vi "Translator.vi"(0 "Input":variant, 11 "error in (no error)":errorcluster) -> (4 "Output":variant, 15 "error out":errorcluster)   [LabVIEW 2014, in "Complex Numbers Static.lvlib"]
doc: "An example of how to create the Translator to convert the LabVIEW VIs to Arduino C code."
uses:
  Complex Numbers Static.lvlib
panel:
  out "Outputs":string[](array[string])
  out "Inputs":string[](array[string])
  out "Output Datatypes":string[](array[string])
  out "Input Datatypes":string[](array[string])
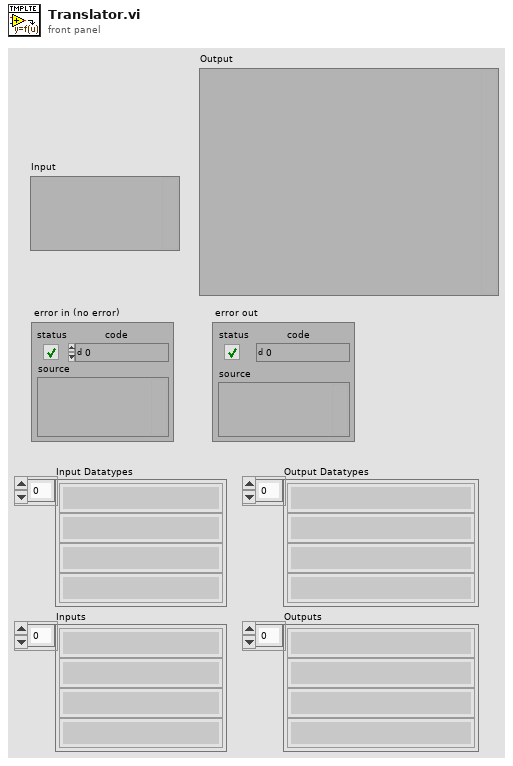
[diagram p1: front panel]
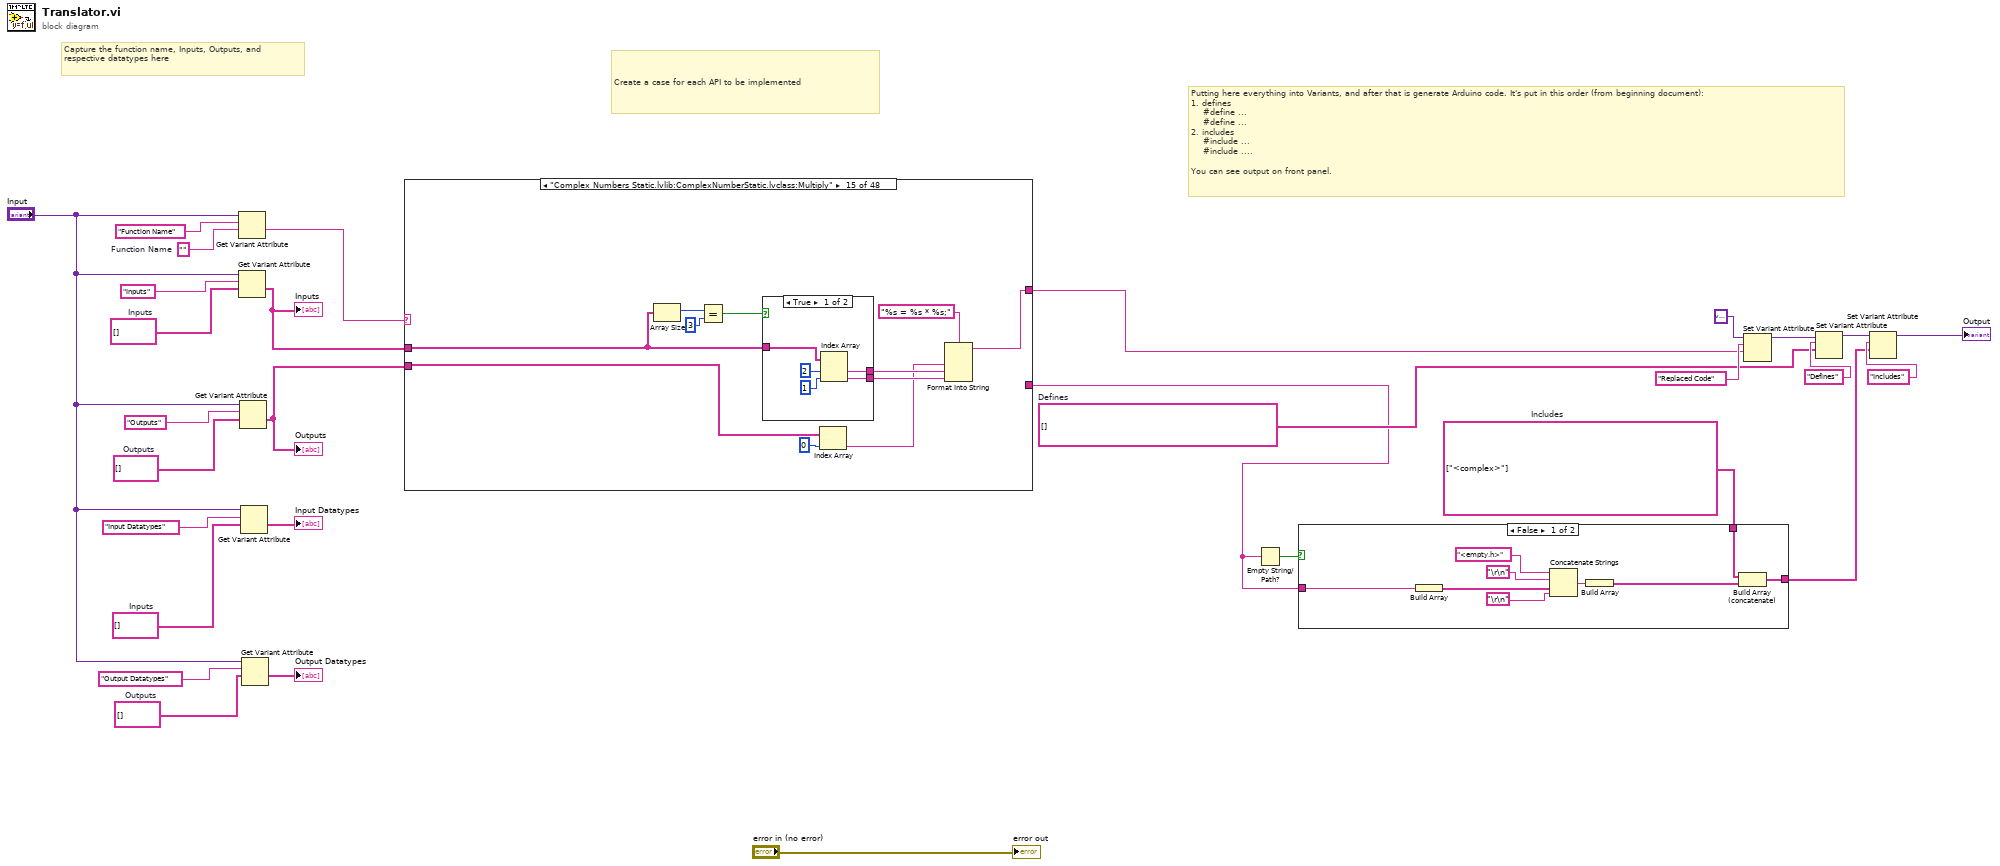
[diagram p0: block diagram]
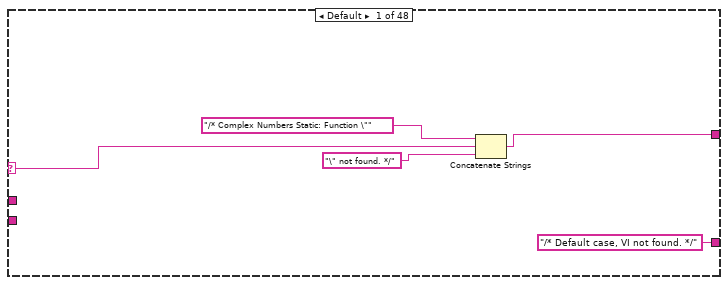
[diagram p3: hidden frame]
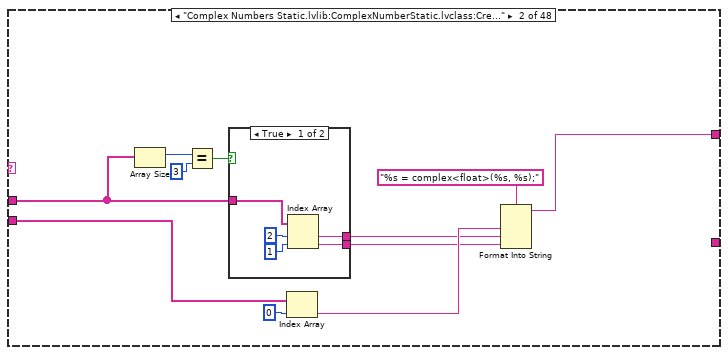
[diagram p4: hidden frame]
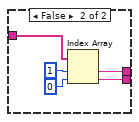
[diagram p5: hidden frame]
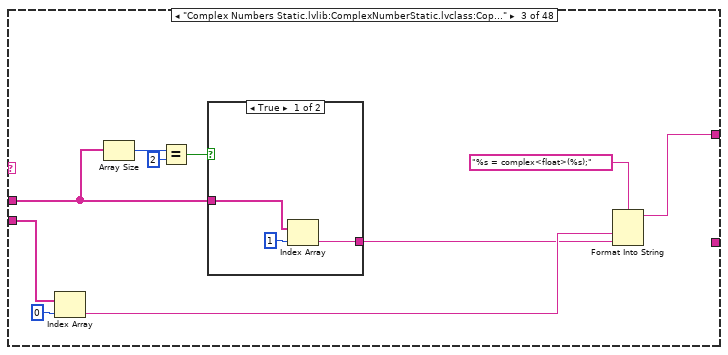
[diagram p6: hidden frame]
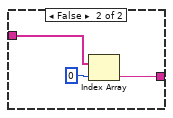
[diagram p7: hidden frame]
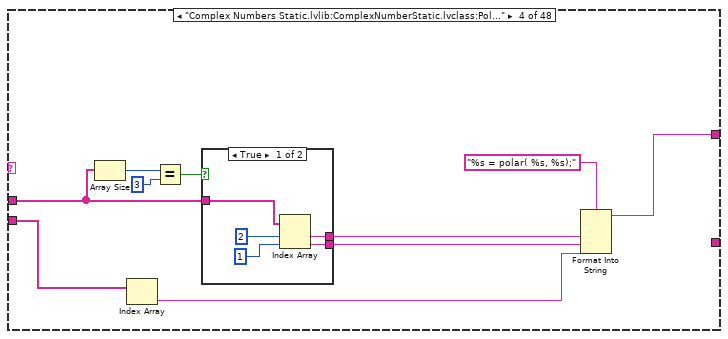
[diagram p8: hidden frame]
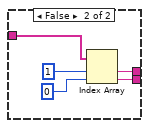
[diagram p9: hidden frame]
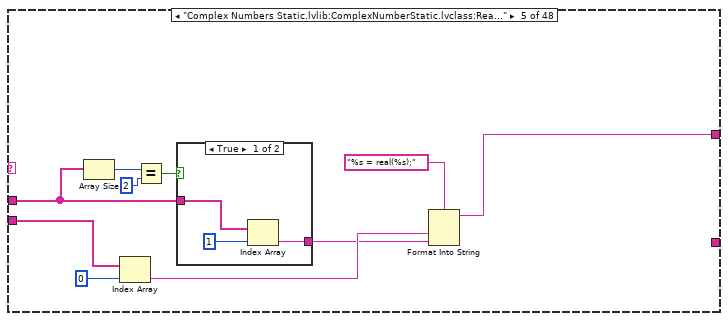
[diagram p10: hidden frame]
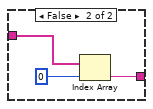
[diagram p11: hidden frame]
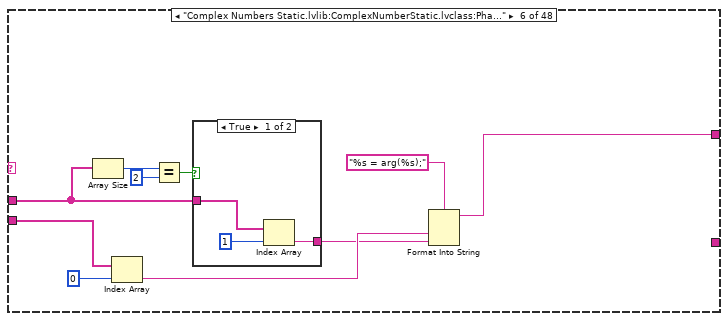
[diagram p12: hidden frame]
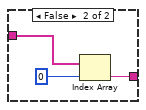
[diagram p13: hidden frame]
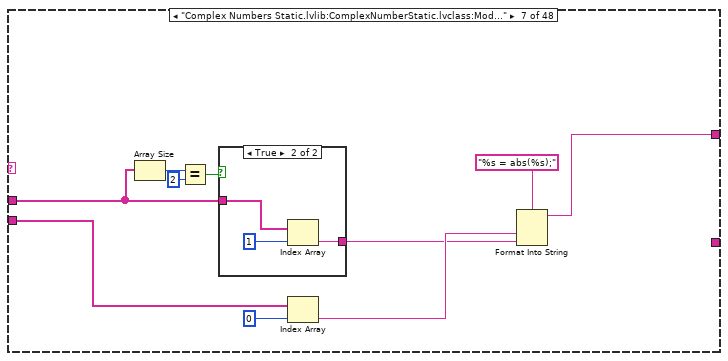
[diagram p14: hidden frame]
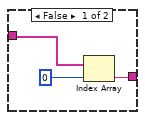
[diagram p15: hidden frame]
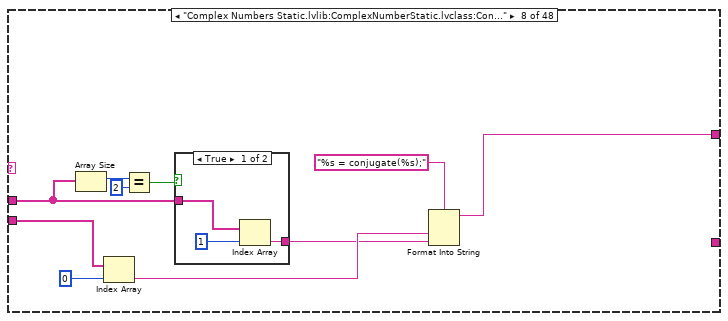
[diagram p16: hidden frame]
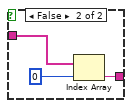
[diagram p17: hidden frame]
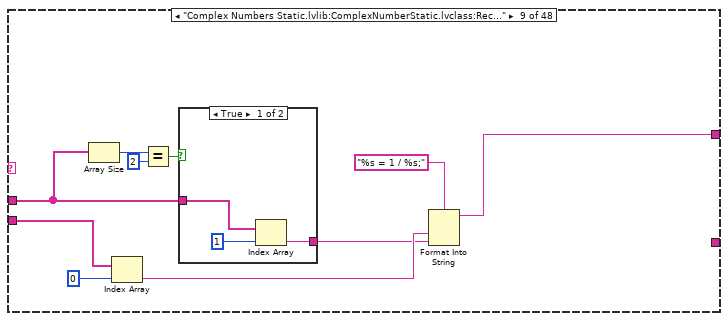
[diagram p18: hidden frame]
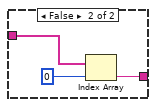
[diagram p19: hidden frame]
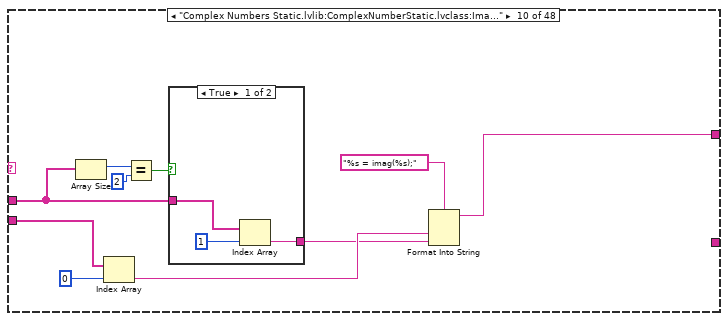
[diagram p20: hidden frame]
diagram:
  w4 = string[] []  # Defines
  w19 = string[] []  # Outputs
  w20 = string[] []  # Inputs
  w1 = string[] ["<complex>"]  # Includes
  w26 = string[] []  # Outputs
  w27 = string[] []  # Inputs
  w28 = ""  # Function Name
  # "Capture the function name, Inputs, Outputs, and respective datatypes here"
  # "Putting here everything into Variants, and after that is generate Arduino code. It's put in this order (from beginning document):\n1. defines\n    #define ...\n    #define ...\n2. includes\n    #include ...\n    #include ....\n\nYou can see output on front panel."
  # "Create a case for each API to be implemented"
  n1 = Get Variant Attribute(Variant="Input", name="Function Name", default value (empty Variant)=w28) -> (value=w10:string)  [unwired: 1 in, 3 out]
  n2 = Get Variant Attribute(Variant="Input", name="Inputs", default value (empty Variant)=w27) -> (value=w9:string[])  [unwired: 1 in, 3 out]
  "Inputs" <- w9
  n3 = Get Variant Attribute(Variant="Input", name="Outputs", default value (empty Variant)=w26) -> (value=w8:string[])  [unwired: 1 in, 3 out]
  "Outputs" <- w8
  n4 = Get Variant Attribute(Variant="Input", name="Input Datatypes", default value (empty Variant)=w20) -> (value=→"Input Datatypes":string[])  [unwired: 1 in, 3 out]
  n5 = Get Variant Attribute(Variant="Input", name="Output Datatypes", default value (empty Variant)=w19) -> (value=→"Output Datatypes":string[])  [unwired: 1 in, 3 out]
  n6 = case shown="\"Complex Numbers Static.lvlib:ComplexNumberStatic.lvclass:Multiply\"" w10 {
    selector: w10 -> [w33 _ _ _ _ _ _ _ _ _ _ _ _ _ _ _ _ _ _ _ _ _ _ _ _ _ _ _ _ _ _ _ _ _ _ _ _ _ _ _ _ _ _ _ _ _ _ _]
    tunnel: w9 -> [_ w37 w57 w74 w94 w112 w128 w142 w158 w174 w191 w197 w218 w240 w260 w281 w302 w325 w339 w356 w377 w393 w410 w426 w445 w461 w478 w493 w509 w525 w541 w557 w573 w589 w605 w623 w637 w654 w670 w685 w701 w717 w733 w749 w766 w782 _ w813]
    tunnel: w8 -> [_ w43 w63 w77 w99 w115 w131 w147 w163 w179 w194 w204 w225 w246 w267 w289 w310 w330 w346 w363 w383 w399 w415 w432 w452 w468 w484 w500 w516 w532 w548 w564 w580 w596 w612 w622 w644 w660 w676 w692 w708 w724 w740 w756 w772 w788 w797 w819]
    tunnel: [w31 w42 w62 w82 w101 w117 w133 w149 w165 w181 w193 w202 w224 w245 w265 w288 w309 w329 w345 w362 w382 w398 w414 w431 w451 w467 w483 w499 w515 w531 w547 w563 w579 w595 w611 w621 w643 w659 w675 w691 w707 w723 w739 w755 w771 w787 w803 w818] -> w7
    tunnel: ["/* Default case, VI not found. */" ("name") _ _ _ _ _ _ _ _ _ _ _ _ _ _ _ _ _ _ _ _ _ _ _ _ _ _ _ _ _ _ _ _ _ _ _ _ _ _ _ _ _ _ _ _ _ _ _] -> w3
    frame Default {
      n7 = Concatenate Strings("/* Complex Numbers Static: Function \"" ("string"), w33, "\" not found. */" ("string")) -> (w31:string)
    }
    frame "Complex Numbers Static.lvlib:ComplexNumberStatic.lvclass:Create" {
      n8 = Array Size(array=w37) -> (size(s)=w38:i32)
      n9 = Equal?(x=w38, y=3) -> (x = y?=w39:bool)
      n10 = case shown="True" w39 {
        tunnel: w37 -> [w50 w55]
        tunnel: [w49 w54] -> w41
        tunnel: [w48 w53] -> w40
        frame True {
          n11 = Index Array(array=w50, index #1=2 ("index"), index #2=1 ("index")) -> (element #1=w49:string, element #2=w48:string)
        }
        frame False {
          n12 = Index Array(array=w55, index #1=1 ("index"), index #2=0 ("index")) -> (element #1=w54:string, element #2=w53:string)
        }
      }
      n13 = Index Array(array=w43, index=0) -> (element=w45:string)
      n14 = Format Into String(format string="%s = complex<float>(%s, %s);", w45, w41, w40) -> (resulting string=w42:string)  [unwired: 2 in, 1 out]
    }
    frame "Complex Numbers Static.lvlib:ComplexNumberStatic.lvclass:Copy" {
      n15 = Index Array(array=w63, index=0) -> (element=w65:string)
      n16 = Array Size(array=w57) -> (size(s)=w60:i32)
      n17 = Equal?(x=w60, y=2) -> (x = y?=w59:bool)
      n18 = case shown="True" w59 {
        tunnel: w57 -> [w68 w71]
        tunnel: [w67 w70] -> w61
        frame True {
          n19 = Index Array(array=w68, index=1) -> (element=w67:string)
        }
        frame False {
          n20 = Index Array(array=w71, index=0) -> (element=w70:string)
        }
      }
      n21 = Format Into String(format string="%s = complex<float>(%s);", w65, w61) -> (resulting string=w62:string)  [unwired: 2 in, 1 out]
    }
    frame "Complex Numbers Static.lvlib:ComplexNumberStatic.lvclass:Polar" {
      n22 = Array Size(array=w74) -> (size(s)=w79:i32)
      n23 = Index Array(array=w77) -> (element=w76:string)  [unwired: 1 in]
      n24 = Equal?(x=w79, y=3) -> (x = y?=w75:bool)
      n25 = case shown="True" w75 {
        tunnel: w74 -> [w86 w91]
        tunnel: [w84 w89] -> w81
        tunnel: [w83 w88] -> w80
        frame True {
          n26 = Index Array(array=w86, index #1=2 ("index"), index #2=1 ("index")) -> (element #1=w84:string, element #2=w83:string)
        }
        frame False {
          n27 = Index Array(array=w91, index #1=1 ("index"), index #2=0 ("index")) -> (element #1=w89:string, element #2=w88:string)
        }
      }
      n28 = Format Into String(format string="%s = polar( %s, %s);", w81, w80, w76) -> (resulting string=w82:string)  [unwired: 2 in, 1 out]
    }
    frame "Complex Numbers Static.lvlib:ComplexNumberStatic.lvclass:Real" {
      n29 = Array Size(array=w94) -> (size(s)=w95:i32)
      n30 = Index Array(array=w99, index=0) -> (element=w98:string)
      n31 = Equal?(x=w95, y=2) -> (x = y?=w96:bool)
      n32 = case shown="True" w96 {
        tunnel: w94 -> [w104 w107]
        tunnel: [w103 w106] -> w97
        frame True {
          n33 = Index Array(array=w104, index=1) -> (element=w103:string)
        }
        frame False {
          n34 = Index Array(array=w107, index=0) -> (element=w106:string)
        }
      }
      n35 = Format Into String(format string="%s = real(%s);", w98, w97) -> (resulting string=w101:string)  [unwired: 2 in, 1 out]
    }
    frame "Complex Numbers Static.lvlib:ComplexNumberStatic.lvclass:Phase" {
      n36 = Array Size(array=w112) -> (size(s)=w110:i32)
      n37 = Index Array(array=w115, index=0) -> (element=w114:string)
      n38 = Equal?(x=w110, y=2) -> (x = y?=w111:bool)
      n39 = case shown="True" w111 {
        tunnel: w112 -> [w120 w123]
        tunnel: [w119 w122] -> w113
        frame True {
          n40 = Index Array(array=w120, index=1) -> (element=w119:string)
        }
        frame False {
          n41 = Index Array(array=w123, index=0) -> (element=w122:string)
        }
      }
      n42 = Format Into String(format string="%s = arg(%s);", w114, w113) -> (resulting string=w117:string)  [unwired: 2 in, 1 out]
    }
    frame "Complex Numbers Static.lvlib:ComplexNumberStatic.lvclass:Modulus" {
      n43 = Array Size(array=w128) -> (size(s)=w127:i32)
      n44 = Equal?(x=w127, y=2) -> (x = y?=w125:bool)
      n45 = case shown="True" w125 {
        tunnel: w128 -> [w136 w139]
        tunnel: [w135 w138] -> w129
        frame False {
          n46 = Index Array(array=w136, index=0) -> (element=w135:string)
        }
        frame True {
          n47 = Index Array(array=w139, index=1) -> (element=w138:string)
        }
      }
      n48 = Index Array(array=w131, index=0) -> (element=w130:string)
      n49 = Format Into String(format string="%s = abs(%s);", w130, w129) -> (resulting string=w133:string)  [unwired: 2 in, 1 out]
    }
    frame "Complex Numbers Static.lvlib:ComplexNumberStatic.lvclass:Conjugate" {
      n50 = Array Size(array=w142) -> (size(s)=w143:i32)
      n51 = Index Array(array=w147, index=0) -> (element=w146:string)
      n52 = Equal?(x=w143, y=2) -> (x = y?=w144:bool)
      n53 = case shown="True" w144 {
        tunnel: w142 -> [w152 w155]
        tunnel: [w151 w154] -> w145
        frame True {
          n54 = Index Array(array=w152, index=1) -> (element=w151:string)
        }
        frame False {
          n55 = Index Array(array=w155, index=0) -> (element=w154:string)
        }
      }
      n56 = Format Into String(format string="%s = conjugate(%s);", w146, w145) -> (resulting string=w149:string)  [unwired: 2 in, 1 out]
    }
    frame "Complex Numbers Static.lvlib:ComplexNumberStatic.lvclass:Reciprocal" {
      n57 = Array Size(array=w158) -> (size(s)=w159:i32)
      n58 = Index Array(array=w163, index=0) -> (element=w162:string)
      n59 = Equal?(x=w159, y=2) -> (x = y?=w160:bool)
      n60 = case shown="True" w160 {
        tunnel: w158 -> [w168 w171]
        tunnel: [w167 w170] -> w161
        frame True {
          n61 = Index Array(array=w168, index=1) -> (element=w167:string)
        }
        frame False {
          n62 = Index Array(array=w171, index=0) -> (element=w170:string)
        }
      }
      n63 = Format Into String(format string="%s = 1 / %s;", w162, w161) -> (resulting string=w165:string)  [unwired: 2 in, 1 out]
    }
    frame "Complex Numbers Static.lvlib:ComplexNumberStatic.lvclass:Imag" {
      n64 = Array Size(array=w174) -> (size(s)=w175:i32)
      n65 = Index Array(array=w179, index=0) -> (element=w178:string)
      n66 = Equal?(x=w175, y=2) -> (x = y?=w176:bool)
      n67 = case shown="True" w176 {
        tunnel: w174 -> [w184 w187]
        tunnel: [w183 w186] -> w177
        frame True {
          n68 = Index Array(array=w184, index=1) -> (element=w183:string)
        }
        frame False {
          n69 = Index Array(array=w187, index=0) -> (element=w186:string)
        }
      }
      n70 = Format Into String(format string="%s = imag(%s);", w178, w177) -> (resulting string=w181:string)  [unwired: 2 in, 1 out]
    }
    frame "Complex Numbers Static.lvlib:ComplexNumberStatic.lvclass:To String" {
      n71 = Index Array(array=w194, index=0) -> (element=w190:string)
      n72 = Index Array(array=w191, index=0) -> (element=w189:string)
      n73 = Format Into String(format string="%s = String( String(real(%s)) + String(\" i*\") + String(imag(%s)));", w190, w189, w189) -> (resulting string=w193:string)  [unwired: 2 in, 1 out]
    }
    frame "Complex Numbers Static.lvlib:ComplexNumberStatic.lvclass:Add" {
      n74 = Array Size(array=w197) -> (size(s)=w200:i32)
      n75 = Equal?(x=w200, y=3) -> (x = y?=w198:bool)
      n76 = case shown="True" w198 {
        tunnel: [w212 w217] -> w207
        tunnel: w197 -> [w209 w214]
        tunnel: [w208 w213] -> w203
        frame True {
          n77 = Index Array(array=w209, index=2) -> (element=w212:string)
          n78 = Index Array(array=w209, index=1) -> (element=w208:string)
        }
        frame False {
          n79 = Index Array(array=w214, index=1) -> (element=w217:string)
          n80 = Index Array(array=w214, index=0) -> (element=w213:string)
        }
      }
      n81 = Index Array(array=w204, index=0) -> (element=w201:string)
      n82 = Format Into String(format string="%s = %s + %s;", w201, w207, w203) -> (resulting string=w202:string)  [unwired: 2 in, 1 out]
    }
    frame "Complex Numbers Static.lvlib:ComplexNumberStatic.lvclass:Subtract" {
      n83 = Index Array(array=w225, index=0) -> (element=w223:string)
      n84 = Array Size(array=w218) -> (size(s)=w220:i32)
      n85 = Equal?(x=w220, y=3) -> (x = y?=w221:bool)
      n86 = case shown="True" w221 {
        tunnel: [w233 w238] -> w228
        tunnel: w218 -> [w231 w236]
        tunnel: [w229 w234] -> w222
        frame True {
          n87 = Index Array(array=w231, index #1=2 ("index"), index #2=1 ("index")) -> (element #1=w233:string, element #2=w229:string)
        }
        frame False {
          n88 = Index Array(array=w236, index #1=1 ("index"), index #2=0 ("index")) -> (element #1=w238:string, element #2=w234:string)
        }
      }
      n89 = Format Into String(format string="%s = %s - %s;", w223, w228, w222) -> (resulting string=w224:string)  [unwired: 2 in, 1 out]
    }
    frame "Complex Numbers Static.lvlib:ComplexNumberStatic.lvclass:Divide" {
      n90 = Index Array(array=w246, index=0) -> (element=w244:string)
      n91 = Array Size(array=w240) -> (size(s)=w241:i32)
      n92 = Equal?(x=w241, y=3) -> (x = y?=w242:bool)
      n93 = case shown="True" w242 {
        tunnel: [w254 w259] -> w249
        tunnel: w240 -> [w252 w257]
        tunnel: [w250 w255] -> w243
        frame True {
          n94 = Index Array(array=w252, index #1=2 ("index"), index #2=1 ("index")) -> (element #1=w254:string, element #2=w250:string)
        }
        frame False {
          n95 = Index Array(array=w257, index #1=1 ("index"), index #2=0 ("index")) -> (element #1=w259:string, element #2=w255:string)
        }
      }
      n96 = Format Into String(format string="%s = %s / %s;", w244, w249, w243) -> (resulting string=w245:string)  [unwired: 2 in, 1 out]
    }
    frame "Complex Numbers Static.lvlib:ComplexNumberStatic.lvclass:Multiply" {
      n97 = Array Size(array=w260) -> (size(s)=w263:i32)
      n98 = Equal?(x=w263, y=3) -> (x = y?=w261:bool)
      n99 = case shown="True" w261 {
        tunnel: [w275 w280] -> w270
        tunnel: w260 -> [w273 w278]
        tunnel: [w271 w276] -> w266
        frame True {
          n100 = Index Array(array=w273, index #1=2 ("index"), index #2=1 ("index")) -> (element #1=w275:string, element #2=w271:string)
        }
        frame False {
          n101 = Index Array(array=w278, index #1=1 ("index"), index #2=0 ("index")) -> (element #1=w280:string, element #2=w276:string)
        }
      }
      n102 = Index Array(array=w267, index=0) -> (element=w264:string)
      n103 = Format Into String(format string="%s = %s * %s;", w264, w270, w266) -> (resulting string=w265:string)  [unwired: 2 in, 1 out]
    }
    frame "Complex Numbers Static.lvlib:ComplexNumberStatic.lvclass:IsEqual" {
      n104 = Array Size(array=w281) -> (size(s)=w284:i32)
      n105 = Equal?(x=w284, y=3) -> (x = y?=w283:bool)
      n106 = case shown="True" w283 {
        tunnel: w281 -> [w295 w300]
        tunnel: [w294 w299] -> w286
        tunnel: [w293 w298] -> w285
        frame True {
          n107 = Index Array(array=w295, index #1=2 ("index"), index #2=1 ("index")) -> (element #1=w294:string, element #2=w293:string)
        }
        frame False {
          n108 = Index Array(array=w300, index #1=1 ("index"), index #2=0 ("index")) -> (element #1=w299:string, element #2=w298:string)
        }
      }
      n109 = Index Array(array=w289, index=0) -> (element=w287:string)
      n110 = Format Into String(format string="%s = (%s == %s);", w287, w286, w285) -> (resulting string=w288:string)  [unwired: 2 in, 1 out]
    }
    frame "Complex Numbers Static.lvlib:ComplexNumberStatic.lvclass:IsNotEqual" {
      n111 = Array Size(array=w302) -> (size(s)=w305:i32)
      n112 = Index Array(array=w310, index=0) -> (element=w308:string)
      n113 = Equal?(x=w305, y=3) -> (x = y?=w303:bool)
      n114 = case shown="True" w303 {
        tunnel: w302 -> [w316 w321]
        tunnel: [w315 w320] -> w307
        tunnel: [w313 w318] -> w306
        frame True {
          n115 = Index Array(array=w316, index #1=2 ("index"), index #2=1 ("index")) -> (element #1=w315:string, element #2=w313:string)
        }
        frame False {
          n116 = Index Array(array=w321, index #1=1 ("index"), index #2=0 ("index")) -> (element #1=w320:string, element #2=w318:string)
        }
      }
      n117 = Format Into String(format string="%s = (%s != %s);", w308, w307, w306) -> (resulting string=w309:string)  [unwired: 2 in, 1 out]
    }
    frame "Complex Numbers Static.lvlib:ComplexNumberStatic.lvclass:Sqr" {
      n118 = Array Size(array=w325) -> (size(s)=w327:i32)
      n119 = Index Array(array=w330, index=0) -> (element=w328:string)
      n120 = Equal?(x=w327, y=2) -> (x = y?=w324:bool)
      n121 = case shown="True" w324 {
        tunnel: w325 -> [w334 w337]
        tunnel: [w333 w336] -> w323
        frame True {
          n122 = Index Array(array=w334, index=1) -> (element=w333:string)
        }
        frame False {
          n123 = Index Array(array=w337, index=0) -> (element=w336:string)
        }
      }
      n124 = Format Into String(format string="%s = %s * %s;", w328, w323, w323) -> (resulting string=w329:string)  [unwired: 2 in, 1 out]
    }
    frame "Complex Numbers Static.lvlib:ComplexNumberStatic.lvclass:Sqrt" {
      n125 = Index Array(array=w346, index=0) -> (element=w344:string)
      n126 = Array Size(array=w339) -> (size(s)=w342:i32)
      n127 = Equal?(x=w342, y=2) -> (x = y?=w340:bool)
      n128 = case shown="True" w340 {
        tunnel: w339 -> [w350 w353]
        tunnel: [w349 w352] -> w343
        frame True {
          n129 = Index Array(array=w350, index=1) -> (element=w349:string)
        }
        frame False {
          n130 = Index Array(array=w353, index=0) -> (element=w352:string)
        }
      }
      n131 = Format Into String(format string="%s = sqrt(%s);", w344, w343) -> (resulting string=w345:string)  [unwired: 2 in, 1 out]
    }
    frame "Complex Numbers Static.lvlib:ComplexNumberStatic.lvclass:Pow" {
      n132 = Index Array(array=w363, index=0) -> (element=w361:string)
      n133 = Array Size(array=w356) -> (size(s)=w357:i32)
      n134 = Equal?(x=w357, y=3) -> (x = y?=w358:bool)
      n135 = case shown="True" w358 {
        tunnel: [w369 w374] -> w360
        tunnel: w356 -> [w368 w373]
        tunnel: [w367 w372] -> w359
        frame True {
          n136 = Index Array(array=w368, index #1=2 ("index"), index #2=1 ("index")) -> (element #1=w369:string, element #2=w367:string)
        }
        frame False {
          n137 = Index Array(array=w373, index #1=1 ("index"), index #2=0 ("index")) -> (element #1=w374:string, element #2=w372:string)
        }
      }
      n138 = Format Into String(format string="%s = pow(%s, %s);", w361, w360, w359) -> (resulting string=w362:string)  [unwired: 2 in, 1 out]
    }
    frame "Complex Numbers Static.lvlib:ComplexNumberStatic.lvclass:Exp" {
      n139 = Index Array(array=w383, index=0) -> (element=w381:string)
      n140 = Array Size(array=w377) -> (size(s)=w378:i32)
      n141 = Equal?(x=w378, y=2) -> (x = y?=w379:bool)
      n142 = case shown="True" w379 {
        tunnel: w377 -> [w386 w390]
        tunnel: [w387 w389] -> w380
        frame False {
          n143 = Index Array(array=w386, index=0) -> (element=w387:string)
        }
        frame True {
          n144 = Index Array(array=w390, index=1) -> (element=w389:string)
        }
      }
      n145 = Format Into String(format string="%s = exp(%s);", w381, w380) -> (resulting string=w382:string)  [unwired: 2 in, 1 out]
    }
    frame "Complex Numbers Static.lvlib:ComplexNumberStatic.lvclass:Log" {
      n146 = Index Array(array=w399, index=0) -> (element=w397:string)
      n147 = Array Size(array=w393) -> (size(s)=w395:i32)
      n148 = Equal?(x=w395, y=2) -> (x = y?=w394:bool)
      n149 = case shown="True" w394 {
        tunnel: w393 -> [w403 w406]
        tunnel: [w402 w405] -> w396
        frame True {
          n150 = Index Array(array=w403, index=1) -> (element=w402:string)
        }
        frame False {
          n151 = Index Array(array=w406, index=0) -> (element=w405:string)
        }
      }
      n152 = Format Into String(format string="%s = log(%s);", w397, w396) -> (resulting string=w398:string)  [unwired: 2 in, 1 out]
    }
    frame "Complex Numbers Static.lvlib:ComplexNumberStatic.lvclass:Log10" {
      n153 = Array Size(array=w410) -> (size(s)=w411:i32)
      n154 = Index Array(array=w415, index=0) -> (element=w413:string)
      n155 = Equal?(x=w411, y=2) -> (x = y?=w409:bool)
      n156 = case shown="True" w409 {
        tunnel: w410 -> [w419 w422]
        tunnel: [w418 w421] -> w412
        frame True {
          n157 = Index Array(array=w419, index=1) -> (element=w418:string)
        }
        frame False {
          n158 = Index Array(array=w422, index=0) -> (element=w421:string)
        }
      }
      n159 = Format Into String(format string="%s = log10(%s);", w413, w412) -> (resulting string=w414:string)  [unwired: 2 in, 1 out]
    }
    frame "Complex Numbers Static.lvlib:ComplexNumberStatic.lvclass:LogN" {
      n160 = Array Size(array=w426) -> (size(s)=w427:i32)
      n161 = Index Array(array=w432, index=0) -> (element=w430:string)
      n162 = Equal?(x=w427, y=2) -> (x = y?=w424:bool)
      n163 = case shown="True" w424 {
        tunnel: [w438 w443] -> w429
        tunnel: w426 -> [w437 w442]
        tunnel: [w436 w441] -> w428
        frame True {
          n164 = Index Array(array=w437, index #1=2 ("index"), index #2=1 ("index")) -> (element #1=w438:string, element #2=w436:string)
        }
        frame False {
          n165 = Index Array(array=w442, index #1=1 ("index"), index #2=0 ("index")) -> (element #1=w443:string, element #2=w441:string)
        }
      }
      n166 = Format Into String(format string="%s = log(%s) / log(%s);", w430, w429, w428) -> (resulting string=w431:string)  [unwired: 2 in, 1 out]
    }
    frame "Complex Numbers Static.lvlib:ComplexNumberStatic.lvclass:Sin" {
      n167 = Index Array(array=w452, index=0) -> (element=w450:string)
      n168 = Array Size(array=w445) -> (size(s)=w448:i32)
      n169 = Equal?(x=w448, y=2) -> (x = y?=w446:bool)
      n170 = case shown="True" w446 {
        tunnel: w445 -> [w456 w459]
        tunnel: [w455 w458] -> w449
        frame True {
          n171 = Index Array(array=w456, index=1) -> (element=w455:string)
        }
        frame False {
          n172 = Index Array(array=w459, index=0) -> (element=w458:string)
        }
      }
      n173 = Format Into String(format string="%s = sin(%s);", w450, w449) -> (resulting string=w451:string)  [unwired: 2 in, 1 out]
    }
    frame "Complex Numbers Static.lvlib:ComplexNumberStatic.lvclass:Cos" {
      n174 = Array Size(array=w461) -> (size(s)=w463:i32)
      n175 = Index Array(array=w468, index=0) -> (element=w466:string)
      n176 = Equal?(x=w463, y=2) -> (x = y?=w464:bool)
      n177 = case shown="True" w464 {
        tunnel: w461 -> [w472 w475]
        tunnel: [w471 w474] -> w465
        frame True {
          n178 = Index Array(array=w472, index=1) -> (element=w471:string)
        }
        frame False {
          n179 = Index Array(array=w475, index=0) -> (element=w474:string)
        }
      }
      n180 = Format Into String(format string="%s = cos(%s);", w466, w465) -> (resulting string=w467:string)  [unwired: 2 in, 1 out]
    }
    frame "Complex Numbers Static.lvlib:ComplexNumberStatic.lvclass:Tan" {
      n181 = Index Array(array=w484, index=0) -> (element=w482:string)
      n182 = Array Size(array=w478) -> (size(s)=w479:i32)
      n183 = Equal?(x=w479, y=2) -> (x = y?=w480:bool)
      n184 = case shown="True" w480 {
        tunnel: w478 -> [w488 w491]
        tunnel: [w487 w490] -> w481
        frame True {
          n185 = Index Array(array=w488, index=1) -> (element=w487:string)
        }
        frame False {
          n186 = Index Array(array=w491, index=0) -> (element=w490:string)
        }
      }
      n187 = Format Into String(format string="%s = tan(%s);", w482, w481) -> (resulting string=w483:string)  [unwired: 2 in, 1 out]
    }
    frame "Complex Numbers Static.lvlib:ComplexNumberStatic.lvclass:Cot" {
      n188 = Index Array(array=w500, index=0) -> (element=w498:string)
      n189 = Array Size(array=w493) -> (size(s)=w496:i32)
      n190 = Equal?(x=w496, y=2) -> (x = y?=w494:bool)
      n191 = case shown="True" w494 {
        tunnel: w493 -> [w504 w507]
        tunnel: [w503 w506] -> w497
        frame True {
          n192 = Index Array(array=w504, index=1) -> (element=w503:string)
        }
        frame False {
          n193 = Index Array(array=w507, index=0) -> (element=w506:string)
        }
      }
      n194 = Format Into String(format string="%s = 1 / tan(%s);", w498, w497) -> (resulting string=w499:string)  [unwired: 2 in, 1 out]
    }
    frame "Complex Numbers Static.lvlib:ComplexNumberStatic.lvclass:Asin" {
      n195 = Index Array(array=w516, index=0) -> (element=w514:string)
      n196 = Array Size(array=w509) -> (size(s)=w512:i32)
      n197 = Equal?(x=w512, y=2) -> (x = y?=w510:bool)
      n198 = case shown="True" w510 {
        tunnel: w509 -> [w520 w523]
        tunnel: [w519 w522] -> w513
        frame True {
          n199 = Index Array(array=w520, index=1) -> (element=w519:string)
        }
        frame False {
          n200 = Index Array(array=w523, index=0) -> (element=w522:string)
        }
      }
      n201 = Format Into String(format string="%s = asin(%s);", w514, w513) -> (resulting string=w515:string)  [unwired: 2 in, 1 out]
    }
    frame "Complex Numbers Static.lvlib:ComplexNumberStatic.lvclass:Acos" {
      n202 = Array Size(array=w525) -> (size(s)=w528:i32)
      n203 = Index Array(array=w532, index=0) -> (element=w530:string)
      n204 = Equal?(x=w528, y=2) -> (x = y?=w526:bool)
      n205 = case shown="True" w526 {
        tunnel: w525 -> [w536 w539]
        tunnel: [w535 w538] -> w529
        frame True {
          n206 = Index Array(array=w536, index=1) -> (element=w535:string)
        }
        frame False {
          n207 = Index Array(array=w539, index=0) -> (element=w538:string)
        }
      }
      n208 = Format Into String(format string="%s = acos(%s);", w530, w529) -> (resulting string=w531:string)  [unwired: 2 in, 1 out]
    }
    frame "Complex Numbers Static.lvlib:ComplexNumberStatic.lvclass:Atan" {
      n209 = Array Size(array=w541) -> (size(s)=w544:i32)
      n210 = Index Array(array=w548, index=0) -> (element=w546:string)
      n211 = Equal?(x=w544, y=2) -> (x = y?=w542:bool)
      n212 = case shown="True" w542 {
        tunnel: w541 -> [w552 w555]
        tunnel: [w551 w554] -> w545
        frame True {
          n213 = Index Array(array=w552, index=1) -> (element=w551:string)
        }
        frame False {
          n214 = Index Array(array=w555, index=0) -> (element=w554:string)
        }
      }
      n215 = Format Into String(format string="%s = atan(%s);", w546, w545) -> (resulting string=w547:string)  [unwired: 2 in, 1 out]
    }
    frame "Complex Numbers Static.lvlib:ComplexNumberStatic.lvclass:Acot" {
      n216 = Array Size(array=w557) -> (size(s)=w560:i32)
      n217 = Index Array(array=w564, index=0) -> (element=w562:string)
      n218 = Equal?(x=w560, y=2) -> (x = y?=w558:bool)
      n219 = case shown="True" w558 {
        tunnel: w557 -> [w568 w571]
        tunnel: [w567 w570] -> w561
        frame True {
          n220 = Index Array(array=w568, index=1) -> (element=w567:string)
        }
        frame False {
          n221 = Index Array(array=w571, index=0) -> (element=w570:string)
        }
      }
      n222 = Format Into String(format string="%s = PI/2 - atan(%s);", w562, w561) -> (resulting string=w563:string)  [unwired: 2 in, 1 out]
    }
    frame "Complex Numbers Static.lvlib:ComplexNumberStatic.lvclass:Csc" {
      n223 = Array Size(array=w573) -> (size(s)=w576:i32)
      n224 = Index Array(array=w580, index=0) -> (element=w578:string)
      n225 = Equal?(x=w576, y=2) -> (x = y?=w574:bool)
      n226 = case shown="True" w574 {
        tunnel: w573 -> [w584 w587]
        tunnel: [w583 w586] -> w577
        frame True {
          n227 = Index Array(array=w584, index=1) -> (element=w583:string)
        }
        frame False {
          n228 = Index Array(array=w587, index=0) -> (element=w586:string)
        }
      }
      n229 = Format Into String(format string="%s = 1 / sin(%s);", w578, w577) -> (resulting string=w579:string)  [unwired: 2 in, 1 out]
    }
    frame "Complex Numbers Static.lvlib:ComplexNumberStatic.lvclass:Sec" {
      n230 = Array Size(array=w589) -> (size(s)=w592:i32)
      n231 = Index Array(array=w596, index=0) -> (element=w594:string)
      n232 = Equal?(x=w592, y=2) -> (x = y?=w590:bool)
      n233 = case shown="True" w590 {
        tunnel: w589 -> [w600 w603]
        tunnel: [w599 w602] -> w593
        frame True {
          n234 = Index Array(array=w600, index=1) -> (element=w599:string)
        }
        frame False {
          n235 = Index Array(array=w603, index=0) -> (element=w602:string)
        }
      }
      n236 = Format Into String(format string="%s = 1 / cos(%s);", w594, w593) -> (resulting string=w595:string)  [unwired: 2 in, 1 out]
    }
    frame "Complex Numbers Static.lvlib:ComplexNumberStatic.lvclass:Acsc" {
      n237 = Array Size(array=w605) -> (size(s)=w608:i32)
      n238 = Index Array(array=w612, index=0) -> (element=w610:string)
      n239 = Equal?(x=w608, y=2) -> (x = y?=w606:bool)
      n240 = case shown="True" w606 {
        tunnel: w605 -> [w616 w619]
        tunnel: [w615 w618] -> w609
        frame True {
          n241 = Index Array(array=w616, index=1) -> (element=w615:string)
        }
        frame False {
          n242 = Index Array(array=w619, index=0) -> (element=w618:string)
        }
      }
      n243 = Format Into String(format string="%s = asin(1/%s);", w610, w609) -> (resulting string=w611:string)  [unwired: 2 in, 1 out]
    }
    frame "Complex Numbers Static.lvlib:ComplexNumberStatic.lvclass:Asec" {
      n244 = Array Size(array=w623) -> (size(s)=w626:i32)
      n245 = Index Array(array=w622, index=0) -> (element=w628:string)
      n246 = Equal?(x=w626, y=2) -> (x = y?=w624:bool)
      n247 = case shown="True" w624 {
        tunnel: w623 -> [w632 w635]
        tunnel: [w631 w634] -> w627
        frame True {
          n248 = Index Array(array=w632, index=1) -> (element=w631:string)
        }
        frame False {
          n249 = Index Array(array=w635, index=0) -> (element=w634:string)
        }
      }
      n250 = Format Into String(format string="%s = acos(1/%s);", w628, w627) -> (resulting string=w621:string)  [unwired: 2 in, 1 out]
    }
    frame "Complex Numbers Static.lvlib:ComplexNumberStatic.lvclass:Sinh" {
      n251 = Index Array(array=w644, index=0) -> (element=w642:string)
      n252 = Array Size(array=w637) -> (size(s)=w639:i32)
      n253 = Equal?(x=w639, y=2) -> (x = y?=w638:bool)
      n254 = case shown="True" w638 {
        tunnel: w637 -> [w648 w651]
        tunnel: [w647 w650] -> w641
        frame True {
          n255 = Index Array(array=w648, index=1) -> (element=w647:string)
        }
        frame False {
          n256 = Index Array(array=w651, index=0) -> (element=w650:string)
        }
      }
      n257 = Format Into String(format string="%s = sinh(%s);", w642, w641) -> (resulting string=w643:string)  [unwired: 2 in, 1 out]
    }
    frame "Complex Numbers Static.lvlib:ComplexNumberStatic.lvclass:Cosh" {
      n258 = Array Size(array=w654) -> (size(s)=w656:i32)
      n259 = Index Array(array=w660, index=0) -> (element=w658:string)
      n260 = Equal?(x=w656, y=2) -> (x = y?=w653:bool)
      n261 = case shown="True" w653 {
        tunnel: w654 -> [w664 w667]
        tunnel: [w663 w666] -> w657
        frame True {
          n262 = Index Array(array=w664, index=1) -> (element=w663:string)
        }
        frame False {
          n263 = Index Array(array=w667, index=0) -> (element=w666:string)
        }
      }
      n264 = Format Into String(format string="%s = cosh(%s);", w658, w657) -> (resulting string=w659:string)  [unwired: 2 in, 1 out]
    }
    frame "Complex Numbers Static.lvlib:ComplexNumberStatic.lvclass:Tanh" {
      n265 = Index Array(array=w676, index=0) -> (element=w674:string)
      n266 = Array Size(array=w670) -> (size(s)=w673:i32)
      n267 = Equal?(x=w673, y=2) -> (x = y?=w671:bool)
      n268 = case shown="True" w671 {
        tunnel: w670 -> [w680 w683]
        tunnel: [w679 w682] -> w669
        frame True {
          n269 = Index Array(array=w680, index=1) -> (element=w679:string)
        }
        frame False {
          n270 = Index Array(array=w683, index=0) -> (element=w682:string)
        }
      }
      n271 = Format Into String(format string="%s = tanh(%s);", w674, w669) -> (resulting string=w675:string)  [unwired: 2 in, 1 out]
    }
    frame "Complex Numbers Static.lvlib:ComplexNumberStatic.lvclass:Asinh" {
      n272 = Index Array(array=w692, index=0) -> (element=w690:string)
      n273 = Array Size(array=w685) -> (size(s)=w689:i32)
      n274 = Equal?(x=w689, y=2) -> (x = y?=w687:bool)
      n275 = case shown="True" w687 {
        tunnel: w685 -> [w696 w699]
        tunnel: [w695 w698] -> w686
        frame True {
          n276 = Index Array(array=w696, index=1) -> (element=w695:string)
        }
        frame False {
          n277 = Index Array(array=w699, index=0) -> (element=w698:string)
        }
      }
      n278 = Format Into String(format string="%s = asinh(%s);", w690, w686) -> (resulting string=w691:string)  [unwired: 2 in, 1 out]
    }
    frame "Complex Numbers Static.lvlib:ComplexNumberStatic.lvclass:Acosh" {
      n279 = Index Array(array=w708, index=0) -> (element=w706:string)
      n280 = Array Size(array=w701) -> (size(s)=w705:i32)
      n281 = Equal?(x=w705, y=2) -> (x = y?=w703:bool)
      n282 = case shown="True" w703 {
        tunnel: w701 -> [w712 w715]
        tunnel: [w711 w714] -> w702
        frame True {
          n283 = Index Array(array=w712, index=1) -> (element=w711:string)
        }
        frame False {
          n284 = Index Array(array=w715, index=0) -> (element=w714:string)
        }
      }
      n285 = Format Into String(format string="%s = acosh(%s);", w706, w702) -> (resulting string=w707:string)  [unwired: 2 in, 1 out]
    }
    frame "Complex Numbers Static.lvlib:ComplexNumberStatic.lvclass:Atanh" {
      n286 = Index Array(array=w724, index=0) -> (element=w722:string)
      n287 = Array Size(array=w717) -> (size(s)=w721:i32)
      n288 = Equal?(x=w721, y=2) -> (x = y?=w719:bool)
      n289 = case shown="True" w719 {
        tunnel: w717 -> [w728 w731]
        tunnel: [w727 w730] -> w718
        frame True {
          n290 = Index Array(array=w728, index=1) -> (element=w727:string)
        }
        frame False {
          n291 = Index Array(array=w731, index=0) -> (element=w730:string)
        }
      }
      n292 = Format Into String(format string="%s = atanh(%s);", w722, w718) -> (resulting string=w723:string)  [unwired: 2 in, 1 out]
    }
    frame "Complex Numbers Static.lvlib:ComplexNumberStatic.lvclass:Sech" {
      n293 = Array Size(array=w733) -> (size(s)=w737:i32)
      n294 = Index Array(array=w740, index=0) -> (element=w738:string)
      n295 = Equal?(x=w737, y=2) -> (x = y?=w735:bool)
      n296 = case shown="True" w735 {
        tunnel: w733 -> [w744 w747]
        tunnel: [w743 w746] -> w734
        frame True {
          n297 = Index Array(array=w744, index=1) -> (element=w743:string)
        }
        frame False {
          n298 = Index Array(array=w747, index=0) -> (element=w746:string)
        }
      }
      n299 = Format Into String(format string="%s = 1 / cosh(%s);", w738, w734) -> (resulting string=w739:string)  [unwired: 2 in, 1 out]
    }
    frame "Complex Numbers Static.lvlib:ComplexNumberStatic.lvclass:Csch" {
      n300 = Array Size(array=w749) -> (size(s)=w753:i32)
      n301 = Index Array(array=w756, index=0) -> (element=w754:string)
      n302 = Equal?(x=w753, y=2) -> (x = y?=w751:bool)
      n303 = case shown="True" w751 {
        tunnel: w749 -> [w760 w763]
        tunnel: [w759 w762] -> w750
        frame True {
          n304 = Index Array(array=w760, index=1) -> (element=w759:string)
        }
        frame False {
          n305 = Index Array(array=w763, index=0) -> (element=w762:string)
        }
      }
      n306 = Format Into String(format string="%s = 1 / sinh(%s);", w754, w750) -> (resulting string=w755:string)  [unwired: 2 in, 1 out]
    }
    frame "Complex Numbers Static.lvlib:ComplexNumberStatic.lvclass:Coth" {
      n307 = Array Size(array=w766) -> (size(s)=w769:i32)
      n308 = Index Array(array=w772, index=0) -> (element=w770:string)
      n309 = Equal?(x=w769, y=2) -> (x = y?=w767:bool)
      n310 = case shown="True" w767 {
        tunnel: w766 -> [w776 w779]
        tunnel: [w775 w778] -> w765
        frame True {
          n311 = Index Array(array=w776, index=1) -> (element=w775:string)
        }
        frame False {
          n312 = Index Array(array=w779, index=0) -> (element=w778:string)
        }
      }
      n313 = Format Into String(format string="%s = cosh(%s) / sinh(%s);", w770, w765, w765) -> (resulting string=w771:string)  [unwired: 2 in, 1 out]
    }
    frame "Complex Numbers Static.lvlib:ComplexNumberStatic.lvclass:Asech" {
      n314 = Index Array(array=w788, index=0) -> (element=w786:string)
      n315 = Array Size(array=w782) -> (size(s)=w785:i32)
      n316 = Equal?(x=w785, y=2) -> (x = y?=w783:bool)
      n317 = case shown="True" w783 {
        tunnel: w782 -> [w792 w795]
        tunnel: [w791 w794] -> w781
        frame True {
          n318 = Index Array(array=w792, index=1) -> (element=w791:string)
        }
        frame False {
          n319 = Index Array(array=w795, index=0) -> (element=w794:string)
        }
      }
      n320 = Format Into String(format string="%s = acosh(1/%s);", w786, w781) -> (resulting string=w787:string)  [unwired: 2 in, 1 out]
    }
    frame "Complex Numbers Static.lvlib:ComplexNumberStatic.lvclass:Acsch" {
      n321 = Index Array(array=w797, index=0) -> (element=w802:string)
      n322 = Array Size(array=w797) -> (size(s)=w801:i32)
      n323 = Equal?(x=w801, y=2) -> (x = y?=w799:bool)
      n324 = case shown="True" w799 {
        tunnel: w797 -> [w807 w810]
        tunnel: [w806 w809] -> w798
        frame True {
          n325 = Index Array(array=w807, index=1) -> (element=w806:string)
        }
        frame False {
          n326 = Index Array(array=w810, index=0) -> (element=w809:string)
        }
      }
      n327 = Format Into String(format string="%s = asinh(1/%s);", w802, w798) -> (resulting string=w803:string)  [unwired: 2 in, 1 out]
    }
    frame "Complex Numbers Static.lvlib:ComplexNumberStatic.lvclass:Acoth" {
      n328 = Index Array(array=w819, index=0) -> (element=w817:string)
      n329 = Array Size(array=w813) -> (size(s)=w816:i32)
      n330 = Equal?(x=w816, y=2) -> (x = y?=w814:bool)
      n331 = case shown="True" w814 {
        tunnel: w813 -> [w823 w826]
        tunnel: [w822 w825] -> w812
        frame True {
          n332 = Index Array(array=w823, index=1) -> (element=w822:string)
        }
        frame False {
          n333 = Index Array(array=w826, index=0) -> (element=w825:string)
        }
      }
      n334 = Format Into String(format string="%s = atanh(1/%s);", w817, w812) -> (resulting string=w818:string)  [unwired: 2 in, 1 out]
    }
  }
  n335 = Empty String/Path?(string/path=w3) -> (empty?=w5:bool)
  n336 = case shown="False" w5 {
    tunnel: w3 -> [w836 _]
    tunnel: [w829 w837] -> w2
    tunnel: w1 -> [w828 w837]
    frame False {
      n337 = Build Array(w836) -> (w830:string[])
      n338 = Concatenate Strings("<empty.h>" ("string"), "\r\n", w830, "\r\n") -> (w831:string)
      n339 = Build Array(w831) -> (w835:string[])
      n340 = Build Array (concatenate)(w828, w835) -> (w829:string[])
    }
    frame True {
    }
  }
  n341 = Set Variant Attribute(Variant=variant ("variant"), name="Replaced Code", value=w7) -> (Variant out=w13:variant)  [unwired: 1 in, 2 out]
  n342 = Set Variant Attribute(Variant=w13, name="Defines", value=w4) -> (Variant out=w12:variant)  [unwired: 1 in, 2 out]
  n343 = Set Variant Attribute(Variant=w12, name="Includes", value=w2) -> (Variant out=→"Output":variant)  [unwired: 1 in, 2 out]
  "error out" <- "error in (no error)"
